vi "Pulse Measurements (obs).vi"   [LabVIEW 2020, in "NI_MAPro.lvlib"]
uses:
  NI_MAPro.lvlib
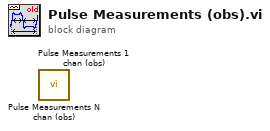
[diagram p0: block diagram]
diagram:
  n1 = call "Pulse Measurements N chan (obs).vi"() -> ()  [unwired: 7 in, 5 out]
  n2 = call "Pulse Measurements 1 chan (obs).vi"() -> ()  [unwired: 7 in, 5 out]
